vi "Automated Sequence Manager.vi"(3 "time [ms]":i32, 4 "Input":T1 {"Emergency State" items=["Closed", "Open"]; "Output Port" items=["DIDO/DO0", "DIDO/DO1", "DIDO/DO2", "DIDO/DO3", "DIDO/DO4", "DIDO/DO5", "DIDO/DO6", "DIDO/DO7", "DIDO/DO8", "DIDO/DO9", "DIDO/DO10", "DIDO/DO11", "DIDO/DO12", "DIDO/DO13", "DIDO/DO14", "DIDO/DO15", "PWM/DO0", "PWM/DO1", "PWM/DO2", "PWM/DO3", "PWM/DO4", "PWM/DO5", "PWM/DO6", "PWM/DO7"]; "Unpowered State" items=["Closed", "Opened"]}) -> (0 "Output":T1 {"Emergency State" items=["Closed", "Open"]; "Output Port" items=["DIDO/DO0", "DIDO/DO1", "DIDO/DO2", "DIDO/DO3", "DIDO/DO4", "DIDO/DO5", "DIDO/DO6", "DIDO/DO7", "DIDO/DO8", "DIDO/DO9", "DIDO/DO10", "DIDO/DO11", "DIDO/DO12", "DIDO/DO13", "DIDO/DO14", "DIDO/DO15", "PWM/DO0", "PWM/DO1", "PWM/DO2", "PWM/DO3", "PWM/DO4", "PWM/DO5", "PWM/DO6", "PWM/DO7"]; "Unpowered State" items=["Closed", "Opened"]}, 1 "Finished":bool)   [LabVIEW 2017]
uses:
  Controls/Manual Control FPGA.ctl
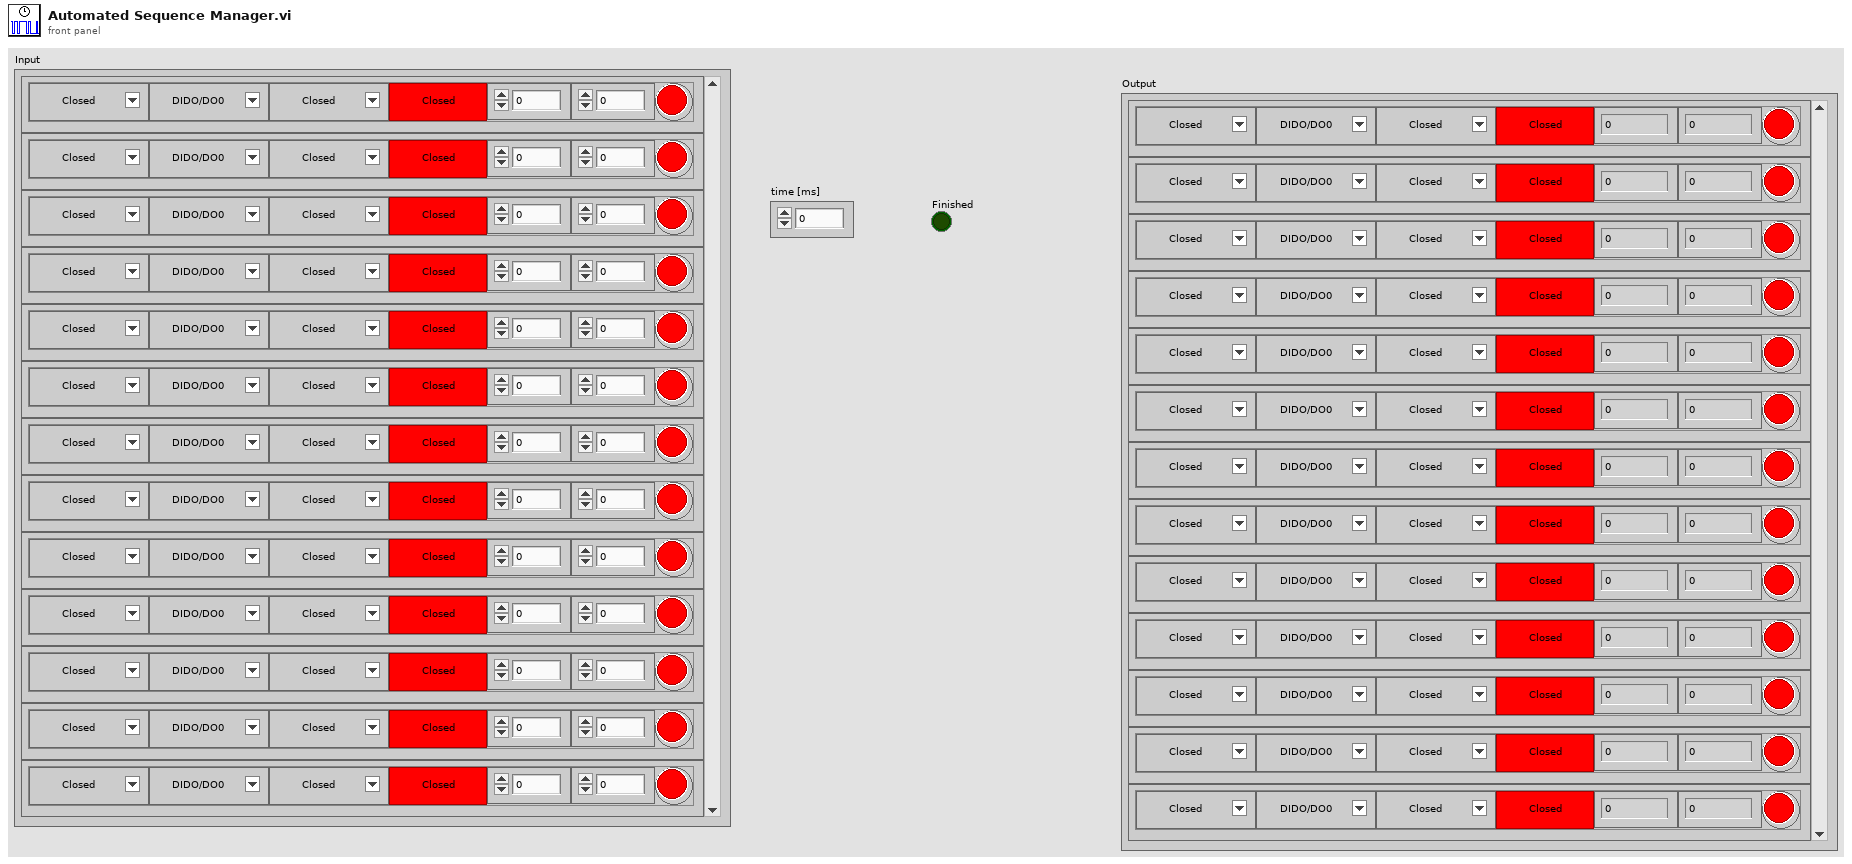
[diagram p1: front panel]
types:
  T1 = typedef "Manual Control FPGA.ctl" = cluster{"Unpowered State":i16, "Output Port":u32, "Emergency State":i16, "Blank Button":bool, "Open Time [ms]":i32, "Close Time [ms]":i32, "Active":bool}[]
  T2 = cluster{"Unpowered State":i16, "Output Port":u32, "Emergency State":i16, "Blank Button":bool, "Open Time [ms]":i32, "Close Time [ms]":i32, "Active":bool}
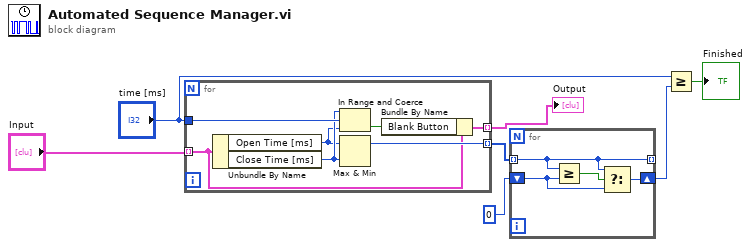
[diagram p0: block diagram]
diagram:
  n1 = for {
    tunnel: "Input" -> [w9] mode=indexing
    tunnel: [w14] -> w4 mode=indexing
    tunnel: "time [ms]" -> [w13]
    tunnel: [w8] -> w1 mode=indexing
    n2 = Unbundle By Name(w9) -> ("Open Time [ms]"=w11:i32, "Close Time [ms]"=w12:i32)
    n3 = In Range and Coerce(upper limit=w12, x=w13, lower limit=w11) -> (In Range?=w10:bool)  [unwired: 1 out]
    n4 = Max & Min(x=w11, y=w12) -> (max(x,y)=w14:i32)  [unwired: 1 out]
    n5 = Bundle By Name(cluster=w9, "Blank Button"=w10) -> (w8:T2)
  }
  "Output" <- w1
  n6 = for {
    tunnel: [w15] -> _ mode=indexing
    shift-right: [w18] -> w5
    shift-left: 0 ("y") -> [w16]
    tunnel: w4 -> [w15] mode=indexing
    n7 = Greater Or Equal?(x=w15, y=w16) -> (x >= y?=w17:bool)
    n8 = Select(t=w15, s=w17, f=w16) -> (s? t:f=w18:i32)
  }
  n9 = Greater Or Equal?(x="time [ms]", y=w5) -> (x >= y?=→"Finished":bool)
